vi "Begin.vi"(8 "error in":errorcluster) -> (0 "error out":errorcluster)   [LabVIEW 2015]
doc: "Called before other user functions, this VI is expected to open initial I/O refnums, load in file data, and do all program initialization. Notice that the <B>error out</B> terminal is simply used for data flow. Wiring it to other structures or subVIs ensures that this VI runs first."
uses:
  <vilib>/Rock Robotics/WPI/DriverStation/WPI_DriverStationRobotMode2.ctl
  <vilib>/Rock Robotics/WPI/Joystick/WPI_JoystickDeviceEnum.ctl
  <vilib>/Rock Robotics/WPI/CAN/TalonSRX/WPI_CANTalonSRX_APIControlMode.ctl
  <vilib>/Rock Robotics/WPI/Solenoid/WPI_SolenoidChannel.ctl
  navX-MXP Library/COMMON/TypeDefs/Value TypeDefs/navX Interface Protocol.ctl
  navX-MXP Library/COMMON/TypeDefs/Value TypeDefs/navX Update Rate.ctl
  Robot Global Data.vi
  <vilib>/Rock Robotics/WPI/MotorControl/WPI_MotorControlOpenCANTalonSRX.vi
  <vilib>/Rock Robotics/WPI/Utilities/WPI_GetSetVariantRefNum.vi
  <vilib>/Rock Robotics/WPI/Solenoid/WPI_SolenoidOpenDouble.vi
  navX-MXP Library/navX-MXP IMU.lvlib
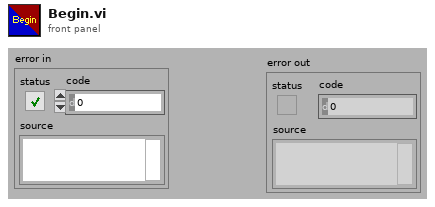
[diagram p1: front panel]
types:
  T1 = typedef "WPI_CANTalonSRX_APIControlMode.ctl" = enum8{"Percent VBus", "Speed", "Position", "Slave", "Unchanged / Invalid", "Voltage Compensation", "Current", "Motion Profile"}
  T2 = typedef "navX-MXP IMU.lvlib/navX Update Rate.ctl" = u8
  T3 = typedef "navX-MXP IMU.lvlib/navX Interface Protocol.ctl" = enum16{"SPI", "I2C", "SERIAL"}
  T4 = typedef "WPI_SolenoidChannel.ctl" = enum8{"Solenoid 0", "Solenoid 1", "Solenoid 2", "Solenoid 3", "Solenoid 4", "Solenoid 5", "Solenoid 6", "Solenoid 7", "Invalid"}
  T5 = typedef "WPI_JoystickDeviceEnum.ctl" = enum16{"USB 0", "USB 1", "USB 2", "USB 3", "USB 4", "USB 5"}
  T6 = typedef "WPI_DriverStationRobotMode2.ctl" = enum16{"Autonomous Disabled", "Autonomous Enabled", "Teleop Disabled", "Teleop Enabled", "Disconnected", "Finish", "Test Disabled", "Test Enabled", "Emergency Stopped"}
  T7 = typedef "WPI_JoystickDevRef.ctl" = cluster{"Device":T5}
  T8 = typedef "WPI_CompressorDevRef.ctl" = cluster{"DevStatus":errorcluster, "Pneumatics Control Module":u8}
  T9 = typedef "WPI_MotorControlDeviceRef.ctl" = cluster{"DeviceStatus":errorcluster, "Type":T10, "PWM":cluster{"PWM Channel":T11, "DeadBand":T12}, "CAN":cluster{"Device Number":u8, "Control Mode":T13, "Semaphore":T14, "Max Vout":dbl, "TalonSRX Control Mode":T1}, "Invert":bool}
  T10 = typedef "WPI_MotorControlType.ctl" = enum16{"PWM", "CAN", "CANTalonSRX"}
  T11 = typedef "FPGA_DIOPWMChannel.ctl" = enum8{"PWM 0", "PWM 1", "PWM 2", "PWM 3", "PWM 4", "PWM 5", "PWM 6", "PWM 7", "PWM 8", "PWM 9", "PWM MXP 0", "PWM MXP 1", "PWM MXP 2", "PWM MXP 3", "PWM MXP 4", "PWM MXP 5", "PWM MXP 6", "PWM MXP 7", "PWM MXP 8", "PWM MXP 9", "Invalid"}
  T12 = typedef "WPI_PWMDeadband.ctl" = cluster{"Name":string, "maxPositivePwm":i32, "minPositivePwm":i32, "centerPwm":i32, "maxNegativePwm":i32, "minNegativePwm":i32, "angularRange":u16}
  T13 = typedef "WPI_CANJaguar_ControlMode.ctl" = enum8{"Percent VBus", "Current", "Speed", "Position", "Voltage"}
  T14 = typedef "Semaphore RefNum" = refnum<k1>
  T15 = typedef "WPI_SolenoidDevRef.ctl" = cluster{"DevStatus":errorcluster, "Pneumatics Control Module":u8, "Forward Solenoid Channel":T4, "Reverse Solenoid Channel":T4}
  T16 = typedef "navX-MXP IMU.lvlib/navX Device TypeDef.ctl" = cluster{"navX Interface Protocol":T3, "navX Interface Protocol TypeDefs":cluster{"SPIDevRef":T17, "I2CDevRef":T19}, "navX System Information":cluster{"Board Information":T21, "Status":T24, "Offsets":T28, "LastSampleTimestamp":dbl, "LastSampleValid":bool}, "navX Common Information":cluster{"Update Rate (4Hz-60Hz)":T2, "refnum name":string, "error":errorcluster, "LastSampleFPGATimestamp":dbl}}
  T17 = typedef "WPI_SPIDevRef.ctl" = cluster{"DevStatus":errorcluster, "Handle":i32, "SPI Bus":T18}
  T18 = typedef "spi_bus.ctl" = enum16{"SPI On-Board, CS0", "SPI On-Board, CS1", "SPI On-Board, CS2", "SPI On-Board, CS3", "SPI MXP", "Invalid"}
  T19 = typedef "WPI_I2CDevRef.ctl" = cluster{"DevStatus":errorcluster, "Device Address":u8, "Handle":i32, "I2C Bus":T20}
  T20 = typedef "i2c_bus.ctl" = enum16{"I2C On-Board", "I2C MXP", "Invalid"}
  T21 = typedef "navX-MXP IMU.lvlib/navX Board Information.ctl" = cluster{"WhoAmI (50 | 0x32)":u8, "Board Revision":u8, "Firmware Major Version":u8, "Firmware Minor Version":u8, "NAVX_BOARD_CAPABILITY":T22, "NAVX_BOARD_YAW_AXIS":T23}
  T22 = typedef "navX-MXP IMU.lvlib/navX NAVX_BOARD_CAPABILITY.ctl" = cluster{"OMNIMOUNT":bool, "YAW_RESET":bool, "VEL_AND_DISP":bool}
  T23 = typedef "navX-MXP IMU.lvlib/navX NAVX_BOARD_YAW_AXIS.ctl" = cluster{"BOARD_YAW_AXIS_UP":bool, "BOARD_YAW_AXIS":u8}
  T24 = typedef "navX-MXP IMU.lvlib/navX Status Data.ctl" = cluster{"Update Rate Hz":u8, "Accelerometer Full-Scale Range":u8, "Gyro Full-Scale Range":u16, "NAVX_OP_STATUS":T25, "NAVX_CAL_STATUS":T26, "NAVX_SELFTEST_STATUS":u8, "NAVX_SENSOR_STATUS":T27}
  T25 = typedef "navX-MXP IMU.lvlib/navX NAVX_OP_STATUS.ctl" = u8
  T26 = typedef "navX-MXP IMU.lvlib/navX NAVX_CAL_STATUS.ctl" = u8
  T27 = typedef "navX-MXP IMU.lvlib/navX NAVX_SENSOR_STATUS.ctl" = cluster{"MOVING":bool, "YAW_STABLE":bool, "MAG_DISTURBANCE":bool, "ALTITUDE_VALID":bool, "SEALEVEL_PRESS_SET":bool, "FUSED_HEADING_VALID":bool}
  T28 = typedef "navX-MXP IMU.lvlib/navX Offsets Data.ctl" = cluster{"Yaw":dbl, "Quat W":dbl, "Quat X":dbl, "Quat Y":dbl, "Quat Z":dbl}
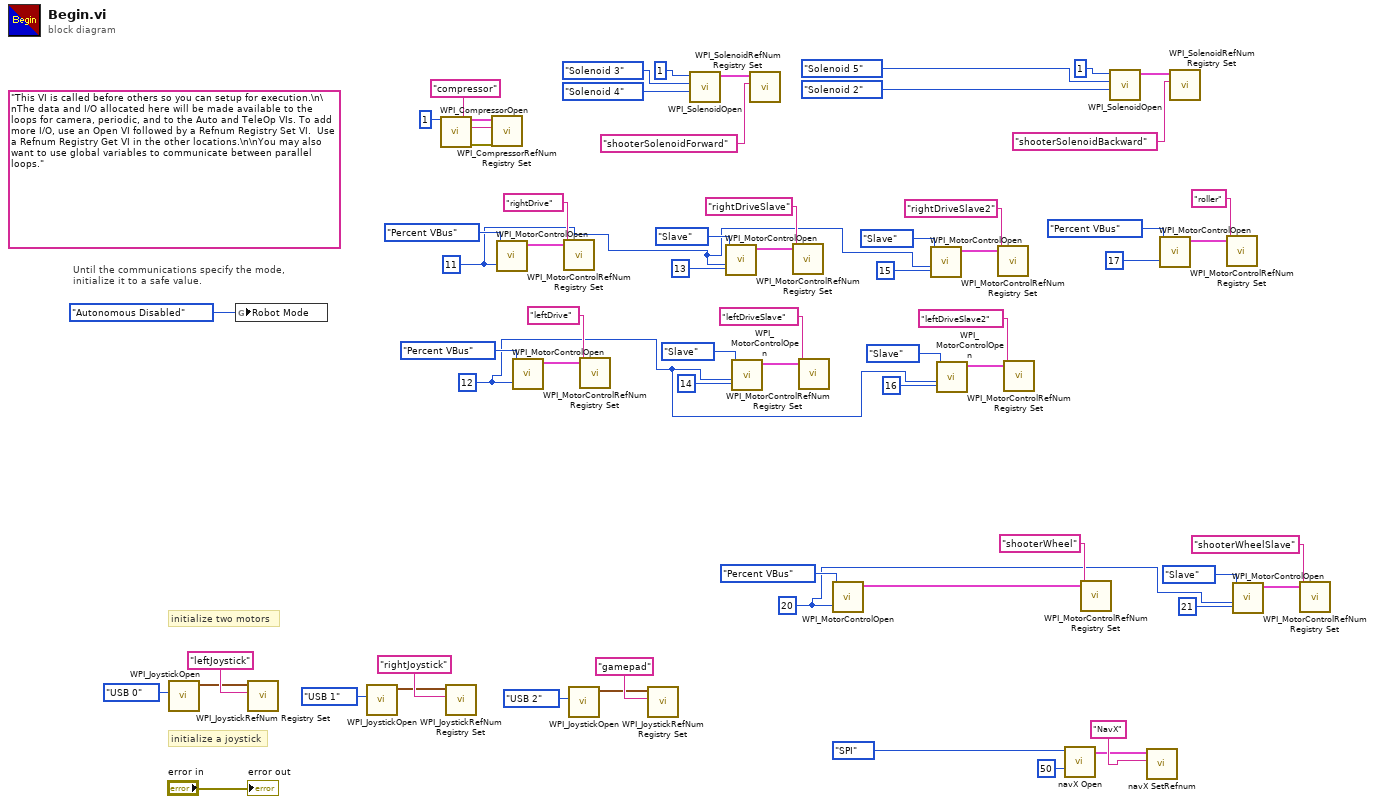
[diagram p0: block diagram]
diagram:
  w29 = u8 20 ("Device Number")
  w2 = u8 12 ("Device Number")
  w1 = u8 11 ("Device Number")
  (unwired) "This VI is called before others so you can setup for execution.\n\nThe data and I/O allocated here will be made available to the loops for camera, periodic, and to the Auto and TeleOp VIs. To add more I/O, use an Open VI followed by a Refnum Registry Set VI.  Use a Refnum Registry Get VI in the other locations.\n\nYou may also want to use global variables to communicate between parallel loops."
  # "initialize a joystick"
  # "Until the communications specify the mode,\ninitialize it to a safe value."
  # "initialize two motors"
  n1 = call <vilib>:"WPI_JoystickOpen.vi"("JoystickDevice"=WPI_JoystickDeviceEnum."USB 0") -> ("JoystickDevRef"=w63:T7)  [unwired: 10 in]
  n2 = global write "Robot Global Data.vi" "Robot Mode"(WPI_DriverStationRobotMode2."Autonomous Disabled" ("Robot Mode")) -> ()
  n3 = call <vilib>:"WPI_JoystickRefNum Registry Set.vi"("refnum name"="leftJoystick", "JoystickDevRef"=w63) -> ()  [unwired: 8 in, 2 out]
  n4 = call <vilib>:"WPI_JoystickOpen.vi"("JoystickDevice"=WPI_JoystickDeviceEnum."USB 1") -> ("JoystickDevRef"=w45:T7)  [unwired: 10 in]
  n5 = call <vilib>:"WPI_CompressorOpen.vi"("Pneumatics Control Module (0)"=u8 1) -> ("CompressorDevRef"=w27:T8, "error out"=w28:errorcluster)  [unwired: 13 in]
  n6 = call <vilib>:"WPI_JoystickRefNum Registry Set.vi"("refnum name"="rightJoystick", "JoystickDevRef"=w45) -> ()  [unwired: 8 in, 2 out]
  n7 = call <vilib>:"WPI_CompressorRefNum Registry Set.vi"("error in (no error)"=w28, "refnum name"="compressor", "CompressorDevRef"=w27) -> ()  [unwired: 7 in, 2 out]
  n8 = call-poly <vilib>:"WPI_MotorControlOpen.vi"("Device Number"=w1, "Control Mode"=WPI_CANTalonSRX_APIControlMode."Percent VBus") -> ("MotorControlDeviceRef"=w60:T9)  [unwired: 8 in, 1 out]
  n9 = call-poly <vilib>:"WPI_MotorControlOpen.vi"("Device Number"=w2, "Control Mode"=WPI_CANTalonSRX_APIControlMode."Percent VBus") -> ("MotorControlDeviceRef"=w53:T9)  [unwired: 8 in, 1 out]
  n10 = call <vilib>:"WPI_MotorControlRefNum Registry Set.vi"("refnum name"="rightDrive", "MotorControlDevRef"=w60) -> ()  [unwired: 8 in, 2 out]
  n11 = call <vilib>:"WPI_JoystickOpen.vi"("JoystickDevice"=WPI_JoystickDeviceEnum."USB 2") -> ("JoystickDevRef"=w42:T7)  [unwired: 10 in]
  n12 = call <vilib>:"WPI_MotorControlRefNum Registry Set.vi"("refnum name"="leftDrive", "MotorControlDevRef"=w53) -> ()  [unwired: 8 in, 2 out]
  n13 = call <vilib>:"WPI_JoystickRefNum Registry Set.vi"("refnum name"="gamepad", "JoystickDevRef"=w42) -> ()  [unwired: 8 in, 2 out]
  n14 = call-poly <vilib>:"WPI_SolenoidOpen.vi"("Reverse Solenoid Channel"=WPI_SolenoidChannel."Solenoid 4", "Forward Solenoid Channel"=WPI_SolenoidChannel."Solenoid 3", "Pneumatics Control Module (0)"=u8 1) -> ("SolenoidDevRef"=w24:T15)  [unwired: 7 in, 1 out]
  n15 = call-poly <vilib>:"WPI_MotorControlOpen.vi"("Master Device Number"=w1, "Device Number"=u8 13, "Control Mode"=WPI_CANTalonSRX_APIControlMode."Slave") -> ("MotorControlDeviceRef"=w57:T9)  [unwired: 7 in, 1 out]
  n16 = call-poly <vilib>:"WPI_MotorControlOpen.vi"("Master Device Number"=w2, "Device Number"=u8 14, "Control Mode"=WPI_CANTalonSRX_APIControlMode."Slave") -> ("MotorControlDeviceRef"=w50:T9)  [unwired: 7 in, 1 out]
  n17 = call <vilib>:"WPI_SolenoidRefNum Registry Set.vi"("refnum name"="shooterSolenoidForward", "SolenoidDevRef"=w24) -> ()  [unwired: 8 in, 2 out]
  n18 = call <vilib>:"WPI_MotorControlRefNum Registry Set.vi"("refnum name"="rightDriveSlave", "MotorControlDevRef"=w57) -> ()  [unwired: 8 in, 2 out]
  n19 = call <vilib>:"WPI_MotorControlRefNum Registry Set.vi"("refnum name"="leftDriveSlave", "MotorControlDevRef"=w50) -> ()  [unwired: 8 in, 2 out]
  n20 = call-poly <vilib>:"WPI_MotorControlOpen.vi"("Device Number"=w29, "Control Mode"=WPI_CANTalonSRX_APIControlMode."Percent VBus") -> ("MotorControlDeviceRef"=w36:T9)  [unwired: 8 in, 1 out]
  n21 = call-poly <vilib>:"WPI_MotorControlOpen.vi"("Master Device Number"=w1, "Device Number"=u8 15, "Control Mode"=WPI_CANTalonSRX_APIControlMode."Slave") -> ("MotorControlDeviceRef"=w3:T9)  [unwired: 7 in, 1 out]
  n22 = call-poly <vilib>:"WPI_MotorControlOpen.vi"("Master Device Number"=w2, "Device Number"=u8 16, "Control Mode"=WPI_CANTalonSRX_APIControlMode."Slave") -> ("MotorControlDeviceRef"=w7:T9)  [unwired: 7 in, 1 out]
  n23 = call <vilib>:"WPI_MotorControlRefNum Registry Set.vi"("refnum name"="rightDriveSlave2", "MotorControlDevRef"=w3) -> ()  [unwired: 8 in, 2 out]
  n24 = call <vilib>:"WPI_MotorControlRefNum Registry Set.vi"("refnum name"="leftDriveSlave2", "MotorControlDevRef"=w7) -> ()  [unwired: 8 in, 2 out]
  n25 = call "navX Open.vi"("Update Rate (4Hz-60Hz)"=T2 50, "navX Interface Protocol"=navX_Interface_Protocol."SPI") -> ("navX Device TypeDef"=w13:T16)  [unwired: 7 in, 2 out]
  n26 = call <vilib>:"WPI_MotorControlRefNum Registry Set.vi"("refnum name"="shooterWheel", "MotorControlDevRef"=w36) -> ()  [unwired: 8 in, 2 out]
  n27 = call-poly <vilib>:"WPI_SolenoidOpen.vi"("Reverse Solenoid Channel"=WPI_SolenoidChannel."Solenoid 2", "Forward Solenoid Channel"=WPI_SolenoidChannel."Solenoid 5", "Pneumatics Control Module (0)"=u8 1) -> ("SolenoidDevRef"=w19:T15)  [unwired: 7 in, 1 out]
  n28 = call "navX SetRefnum.vi"("refnum name"="NavX", "navX Device TypeDef"=w13) -> ()  [unwired: 8 in, 2 out]
  n29 = call-poly <vilib>:"WPI_MotorControlOpen.vi"("Device Number"=u8 17, "Control Mode"=WPI_CANTalonSRX_APIControlMode."Percent VBus") -> ("MotorControlDeviceRef"=w40:T9)  [unwired: 8 in, 1 out]
  n30 = call <vilib>:"WPI_SolenoidRefNum Registry Set.vi"("refnum name"="shooterSolenoidBackward", "SolenoidDevRef"=w19) -> ()  [unwired: 8 in, 2 out]
  n31 = call <vilib>:"WPI_MotorControlRefNum Registry Set.vi"("refnum name"="roller", "MotorControlDevRef"=w40) -> ()  [unwired: 8 in, 2 out]
  n32 = call-poly <vilib>:"WPI_MotorControlOpen.vi"("Master Device Number"=w29, "Device Number"=u8 21, "Control Mode"=WPI_CANTalonSRX_APIControlMode."Slave") -> ("MotorControlDeviceRef"=w33:T9)  [unwired: 7 in, 1 out]
  n33 = call <vilib>:"WPI_MotorControlRefNum Registry Set.vi"("refnum name"="shooterWheelSlave", "MotorControlDevRef"=w33) -> ()  [unwired: 8 in, 2 out]
  "error out" <- "error in"
